vi "ns to um.vi"(9 "number of path lengths (default: 2)":i32=2, 10 "position (ns)":dbl[unit]) -> (2 "position (microns)":dbl[unit])   [LabVIEW 2017]
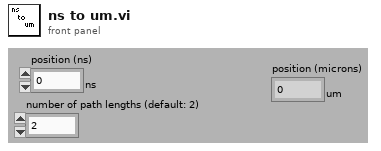
[diagram p1: front panel]
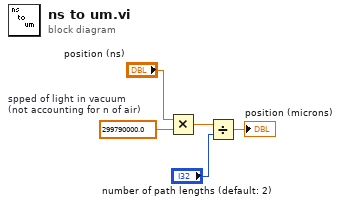
[diagram p0: block diagram]
diagram:
  w5 = dbl[unit] 299790000.0  # spped of light in vacuum (not accounting for n of air)
  n1 = Multiply(x="position (ns)", y=w5) -> (x*y=w3:dbl[unit])
  n2 = Divide(x=w3, y="number of path lengths (default: 2)") -> (x/y=→"position (microns)":dbl[unit])
